vi "Write Config String.vi"(8 "error in (no error)":errorcluster, 10 "RED Channel Settings":T1={"Cooler ON/OFF"=0, "Set temperature"=20.0, "Shutter Mode "=2, "Shutter TTL"=0, "Time to open (ms)"=50.0, "Time to close (ms)"=50.0, "Pre-amplifier gain"=1, "Vertical clock\n  voltage amplitude"=0, "Vertical Shift Speed"=0, "Readout Rate "=0, "Trigger "=0, "Conventional/EM"=1, "Read Mode "=4, "Acquisition Mode "=1, "Exposure Time (s) "=0.0, "Initial Line"=1, "Initial Column"=1, "Final Line"=1, "Final Column"=1, "Horizontal binning"=1, "Vertical binning "=1, "FITS Format"=0, "Image Format"="", "Tiff Position "=1, "Tiff Type"=0, "Image Path"=""} {"Tiff Type" items=["8-bit", "16-bit", "Color"]; "FITS Format" items=["Unsigned 16", "Unsigned 32", "Signed 16", "Signed 32", "Float"]; "Exposure Time (s)" format="%.2f"; "Acquisition Mode" items=["RESERVED", "Single Scan", "Accumulate", "Kinetics", "Fast Kinetics", "Run Til Abort", "RESERVED", "RESERVED", "RESERVED", "RESERVED", "Time Delayed Integration"]; "Read Mode" items=["Full Vertical Binning", "Multi-Track", "Random-Track", "Single-Track", "Image"]; "Conventional/EM" items=["EM Gain", "Conventional"]; "Trigger" items=["Internal", "External", "N/A", "N/A", "N/A", "N/A", "External Start", "External Exposure (bulb)", "N/A", "External FVB EM", "Software", "N/A", "External Charge Shifting"]; "Shutter TTL" items=["TTL Low", "TTL High"]; "Shutter Mode" items=["Fully Auto", "OPEN", "CLOSED"]; "Set temperature" min=-80.0 max=20.0; "Cooler ON/OFF" items=["Cooler OFF", "Cooler ON"]}, 11 "RxTxCamera in":refnum<class "RxTxCamera.lvclass">) -> (0 "error out":errorcluster, 3 "RxTxCamera out":refnum<class "RxTxCamera.lvclass">)   [LabVIEW 2018, in "RxTxCamera.lvclass"]
doc: "Este VI recebe um cluster contendo a configuração da câmera e constrói uma string contendo a configuração e a tag SETUP na primeira linha."
uses:
  RxTxCamera.lvclass
  C:/Users/Cliente/Desktop/Software Echarpe/RxTx/RxTx.lvclass
  RxTxCamera.lvclass/RxTxCamera.ctl
  RxTx/RxTx.lvclass/RxTx.ctl
  Construct String Setup Cam/Construct String Setup Cam.lvclass
  RxTx/RxTx.lvclass
panel:
  # "Set Shutter Configuration"
  # "Timings"
  # "Vertical pixel shift"
  # "(TTL level required to open \nyour external shutter)"
  # "Time to open/close shutter"
  # "Horizontal pixel shift"
  # "Temperature"
  # "Electron Multiplier (EM) Gain"
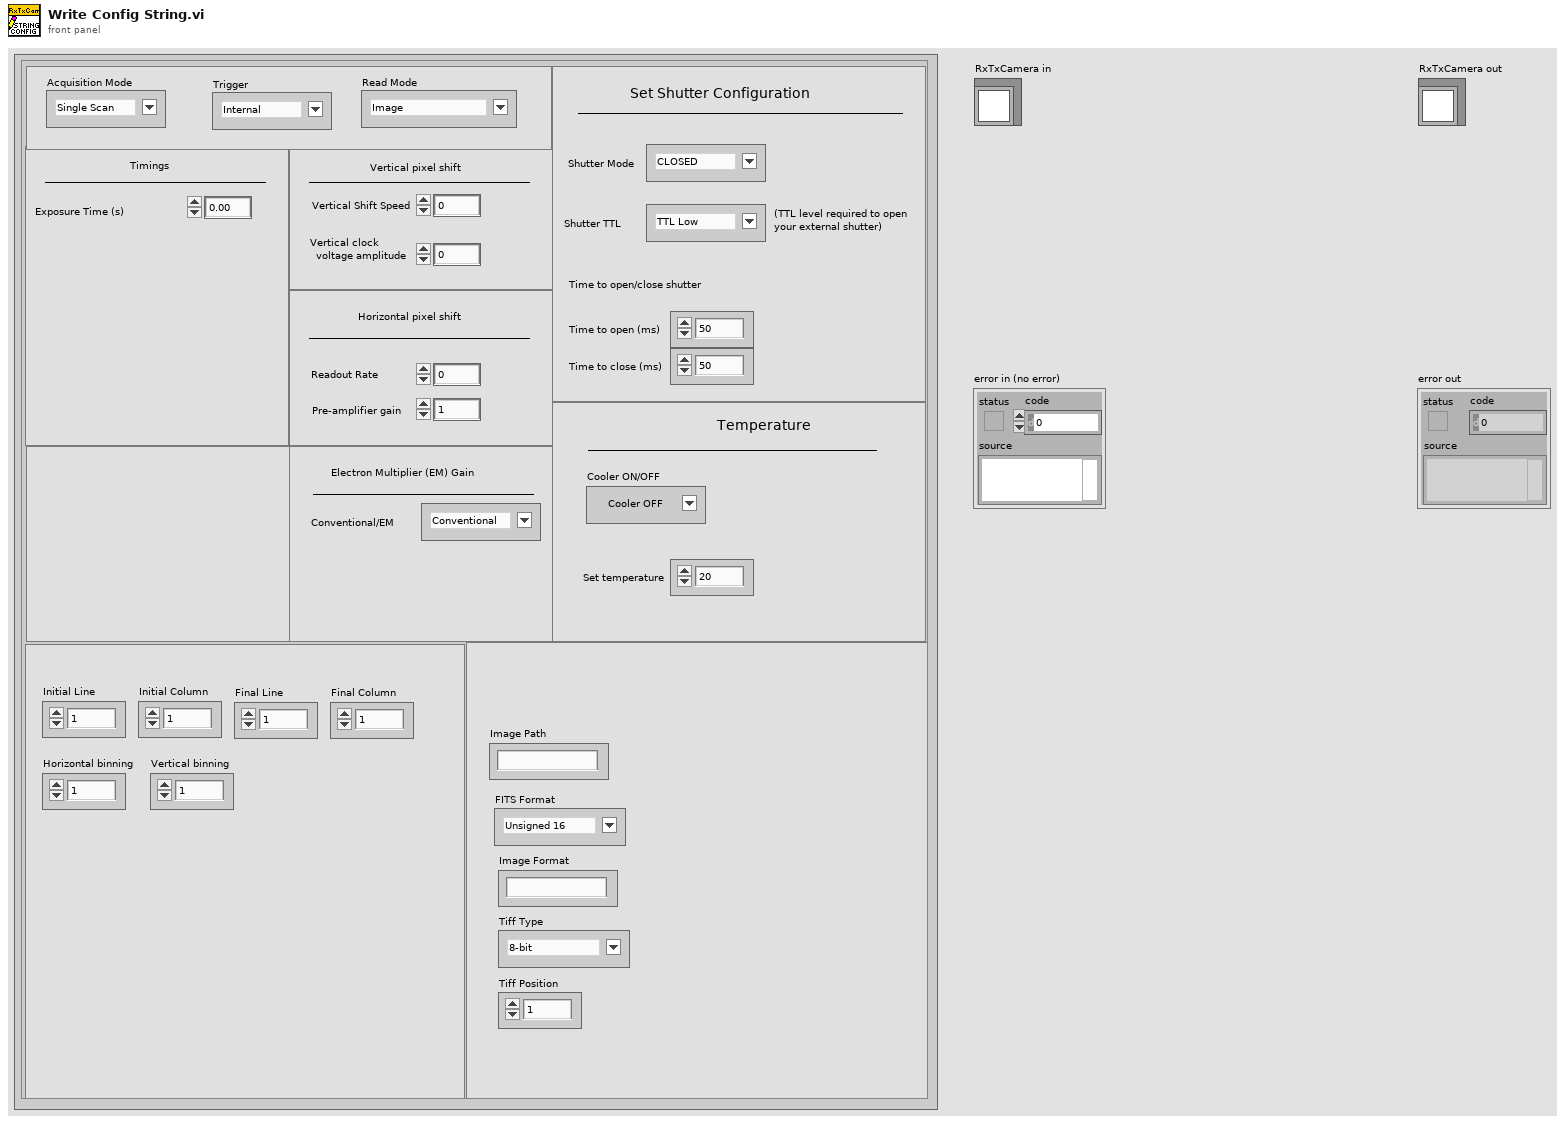
[diagram p1: front panel]
types:
  T1 = cluster{"Cooler ON/OFF":u16, "Set temperature":dbl, "Shutter Mode ":u16, "Shutter TTL":u16, "Time to open (ms)":dbl, "Time to close (ms)":dbl, "Pre-amplifier gain":i32, "Vertical clock\n  voltage amplitude":i32, "Vertical Shift Speed":i32, "Readout Rate ":i32, "Trigger ":u16, "Conventional/EM":i32, "Read Mode ":u16, "Acquisition Mode ":u16, "Exposure Time (s) ":sgl, "Initial Line":i32, "Initial Column":i32, "Final Line":i32, "Final Column":i32, "Horizontal binning":i32, "Vertical binning ":i32, "FITS Format":u16, "Image Format":string, "Tiff Position ":u16, "Tiff Type":u16, "Image Path":string}
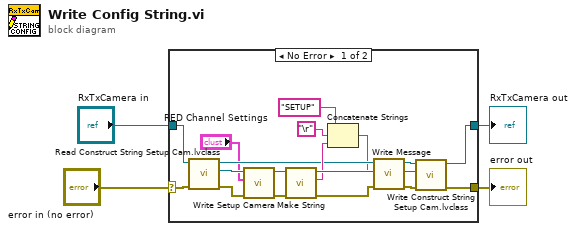
[diagram p0: block diagram]
diagram:
  n1 = case shown="No Error" "error in (no error)" {
    selector: "error in (no error)" -> [w22 w23]
    tunnel: [w20 w23] -> w3
    tunnel: [w19 w24] -> w1
    tunnel: "RxTxCamera in" -> [w21 w24]
    frame No Error {
      n2 = call "Read Construct String Setup Cam.lvclass.vi"("error in (no error)"=w22, "RxTxCamera in"=w21) -> ("error out"=w18:errorcluster, "Construct String Setup Cam.lvclass"=w14:refnum<class "Construct String Setup Cam.lvclass">, "RxTxCamera out"=w8:refnum<class "RxTxCamera.lvclass">)  [unwired: 7 in]
      n3 = call "Write Setup Camera.vi"("error in (no error)"=w18, "RED Channel Settings"="RED Channel Settings", "Construct String Setup Cam in"=w14) -> ("error out"=w17:errorcluster, "Construct String Setup Cam out"=w15:refnum<class "Construct String Setup Cam.lvclass">)  [unwired: 7 in]
      n4 = call "Make String.vi"("error in (no error)"=w17, "Construct String Setup Cam in"=w15) -> ("error out"=w7:errorcluster, "Camera Setup"=w13:string, "Construct String Setup Cam out"=w16:refnum<class "Construct String Setup Cam.lvclass">)  [unwired: 7 in]
      n5 = Concatenate Strings("SETUP", "\r", w13) -> (w6:string)
      n6 = call "Write Message.vi"("error in (no error)"=w7, "Message"=w6, "RxTx in"=w8) -> ("error out"=w10:errorcluster, "RxTx out"=w9:refnum<class "RxTxCamera.lvclass">)  [unwired: 7 in]
      n7 = call "Write Construct String Setup Cam.lvclass.vi"("error in (no error)"=w10, "Construct String Setup Cam.lvclass"=w16, "RxTxCamera in"=w9) -> ("error out"=w20:errorcluster, "RxTxCamera out"=w19:refnum<class "RxTxCamera.lvclass">)  [unwired: 7 in]
    }
    frame Error {
    }
  }
  "error out" <- w3
  "RxTxCamera out" <- w1
